vi "Pre Loop Init.vi"(8 "error in":errorcluster, 11 "Ref In":refnum<vi>) -> (0 "error out":errorcluster, 3 "Event Registration Refnum":refnum<event-registration>)   [LabVIEW 2010, in "Simulated Console.lvlib"]
doc: "This VI performs the pre loop initialisation."
uses:
  Simulated Console.lvlib
  User Events/Controls/UE Abort Action.ctl
  Private Controls/Module Data Cluster.ctl
  Private Controls/Module Action.ctl
  Private Controls/Queue FG Action.ctl
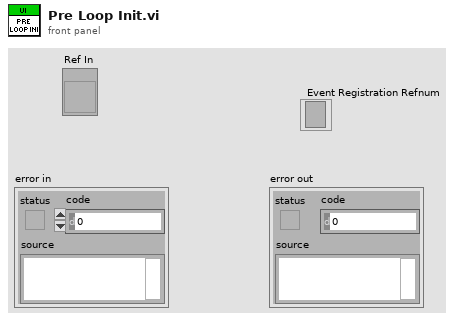
[diagram p1: front panel]
types:
  T1 = typedef "Simulated Console.lvlib/Queue FG Action.ctl" = enum16{"Release", "Get", "Set"}
  T2 = typedef "Simulated Console.lvlib/Module Data Cluster.ctl" = cluster{"Data":variant, "Action":T3}
  T3 = typedef "Simulated Console.lvlib/Module Action.ctl" = enum16{"Error", "Init", "Card", "CancelTransaction", "NewTransaction", "Transaction", "Keypad", "Idle"}
  T4 = typedef "UE Abort Action.ctl" = enum16{"Destroy", "Get", "Create"}
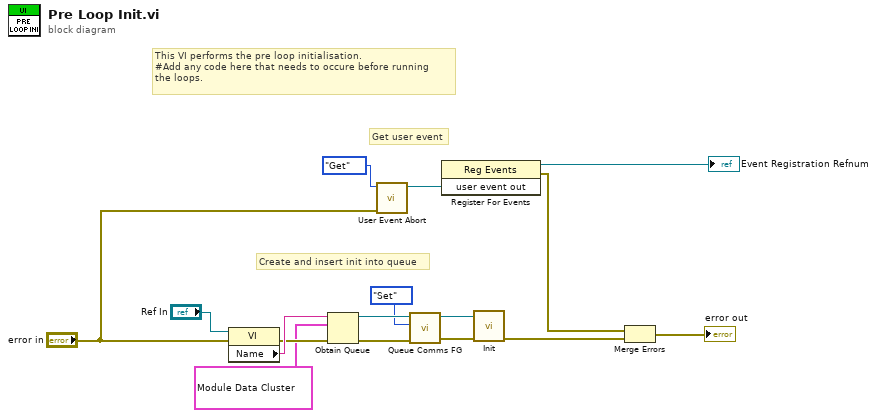
[diagram p0: block diagram]
diagram:
  # "Create and insert init into queue"
  # "Get user event"
  # "This VI performs the pre loop initialisation. \n#Add any code here that needs to occure before running\nthe loops."
  n1 = property on="Property Node" class="VI"(reference="Ref In", error in="error in") -> (error out=w10:errorcluster, "Name"=w12:string)  [unwired: 1 out]
  n2 = Obtain Queue(name (unnamed)=w12, element data type=T2 {"Data"=variant, "Action"=enum."NewTransaction"}, error in (no error)=w10) -> (queue out=w6:refnum<queue>, error out=w4:errorcluster)  [unwired: 2 in, 1 out]
  n3 = call "User Event Abort.vi"("error in"="error in", "Action"=UE_Abort_Action."Get") -> ("user event out"=w15:refnum<user-event>)  [unwired: 8 in, 1 out]
  n4 = call "Queue Comms FG.vi"("error in"=w4, "Action"=Queue_FG_Action."Set", "Queue in"=w6) -> ("error out"=w2:errorcluster, "Queue out"=w3:refnum<queue>)  [unwired: 7 in]
  n5 = register-events(w15) -> (reference out=→"Event Registration Refnum":refnum<event-registration>, error out=w8:errorcluster)  [unwired: 2 in]
  n6 = call "Init.vi"("error in"=w2, "Data"=w3) -> ("error out"=w1:errorcluster)  [unwired: 9 in]
  n7 = Merge Errors(w8, w1) -> (→"error out":errorcluster)
